vi "renameCategory.vi"(8 "error in (no error)":errorcluster, 9 "New Name":string, 10 "Category.lvclass":refnum<class "Category.lvclass">, 11 "Database in":refnum<class "Account History.lvclass">) -> (0 "error out":errorcluster, 3 "Database out":refnum<class "Account History.lvclass">)   [LabVIEW 2018, in "Account History.lvclass"]
uses:
  Account History.lvclass
  Category/Category.lvclass
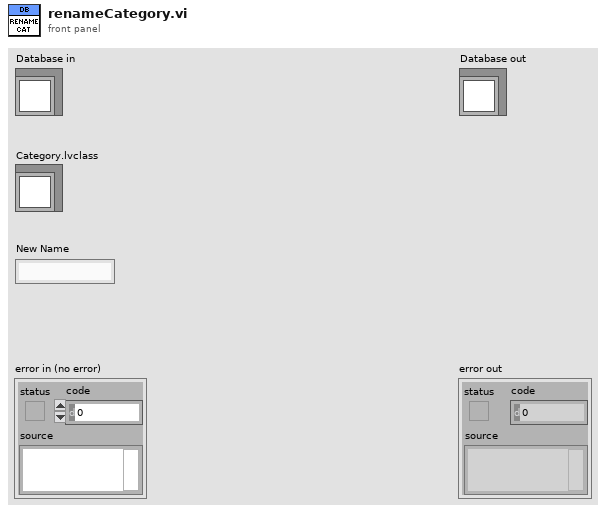
[diagram p1: front panel]
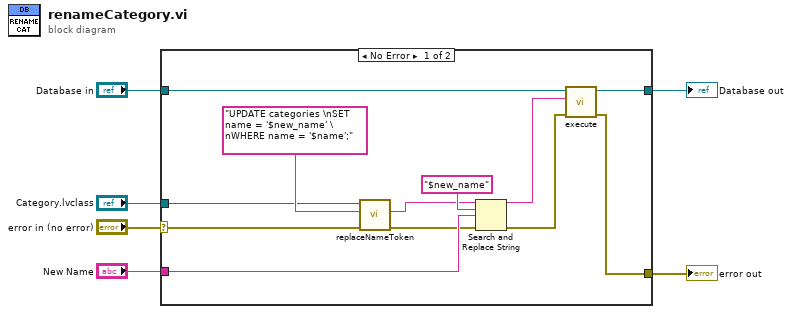
[diagram p0: block diagram]
diagram:
  n1 = case shown="No Error" "error in (no error)" {
    selector: "error in (no error)" -> [w10 w19]
    tunnel: "Database in" -> [w18 w20]
    tunnel: [w17 w20] -> w5
    tunnel: [w16 w19] -> w4
    tunnel: "New Name" -> [w14 _]
    tunnel: "Category.lvclass" -> [w7 _]
    frame No Error {
      n2 = call "replaceNameToken.vi"("error in (no error)"=w10, "Query In"="UPDATE categories \nSET name = '$new_name' \nWHERE name = '$name';", "Category in"=w7) -> ("error out"=w11:errorcluster, "Query Out"=w9:string)  [unwired: 6 in, 1 out]
      n3 = Search and Replace String(input string=w9, search string="$new_name", replace string=w14, error in=w11) -> (result string=w13:string, error out=w12:errorcluster)  [unwired: 4 in, 2 out]
      n4 = call "execute.vi"("error in (no error)"=w12, "SQL query"=w13, "Database in"=w18) -> ("error out"=w16:errorcluster, "Database out"=w17:refnum<class "Account History.lvclass">)  [unwired: 7 in]
    }
    frame Error {
    }
  }
  "error out" <- w4
  "Database out" <- w5
